vi "configure operation.vi"(7 "tag bus configurable plugin module configuration":refnum<class "Modbus Module configuration.lvclass">, 8 "error in":errorcluster, 10 "line item in":T2, 11 "engine configuration":refnum<class "engine configuration.lvclass">) -> (0 "error out":errorcluster, 1 "success":bool, 2 "line item out":T2, 5 "changed":bool)   [LabVIEW 2013, in "Modbus Module editor node.lvclass"]
doc: "Platypus Framework 1.0.1.65\nNI Systems Engineering - National Instruments"
uses:
  Modbus Module editor node.lvclass
  permissions.ctl
  table line.ctl
  module/module channel/Modbus Module Channel.lvclass
  <vilib>/NI/Module Execution Interface/Engine Configuration/engine configuration.lvclass
  module/configuration/Modbus Module configuration.lvclass
  module/module channel/data bank type.ctl
  <vilib>/NI/Tag Bus/tag/tag descriptor.lvclass/tag descriptor.ctl
  <vilib>/NI/Tag Bus Module Framework/channel/TBM channel.lvclass/TBM channel.ctl
  module/module channel/Modbus Module Channel.lvclass/Modbus Module Channel.ctl
  <vilib>/NI/Configuration Framework/serializable configuration/NISE_CEF_serializable configuration.lvclass/NISE_CEF_serializable configuration.ctl
  <vilib>/NI/Tag Bus/tag/Data Type.ctl
  <vilib>/NI/Tag Bus Module Framework/channel/Read channel classification.vi
  module/module channel/Read modbus type.vi
  module/module channel/Read starting address.vi
  module/module channel/Read subindex (bool).vi
  <vilib>/NI/Tag Bus/tag/read data type.vi
  <vilib>/NI/Configuration Framework/serializable configuration/Read UID.vi
  <vilib>/NI/Tag Bus/tag/write data type.vi
  <vilib>/NI/Tag Bus Module Framework/channel/Write channel classification.vi
  module/module channel/Write modbus type.vi
  module/module channel/Write starting address.vi
  module/module channel/Write subindex (bool).vi
  <vilib>/NI/Tag Bus/tag/write tag name.vi
  <vilib>/Utility/LVClass/Get LV Class Name.vi
  <vilib>/NI/Configuration Framework/error generator/NISE_error generator.vi
  <vilib>/NI/Tag Bus/tag/tag descriptor.lvclass
panel:
  in  "Channel Name":string
  out "Alias":string
  out "issues":string
  in  "Tag":i32(listbox)
  in  "Type":i32(listbox)
  in  "Bit/Length":i32 min=0 max=15 step=1
  in  "Address (0 index)":enum16{""}(ring)
  in  "modbus bank":T1
  in  "cancel":bool
  in  "ok":bool
  in  "Access Type":T3
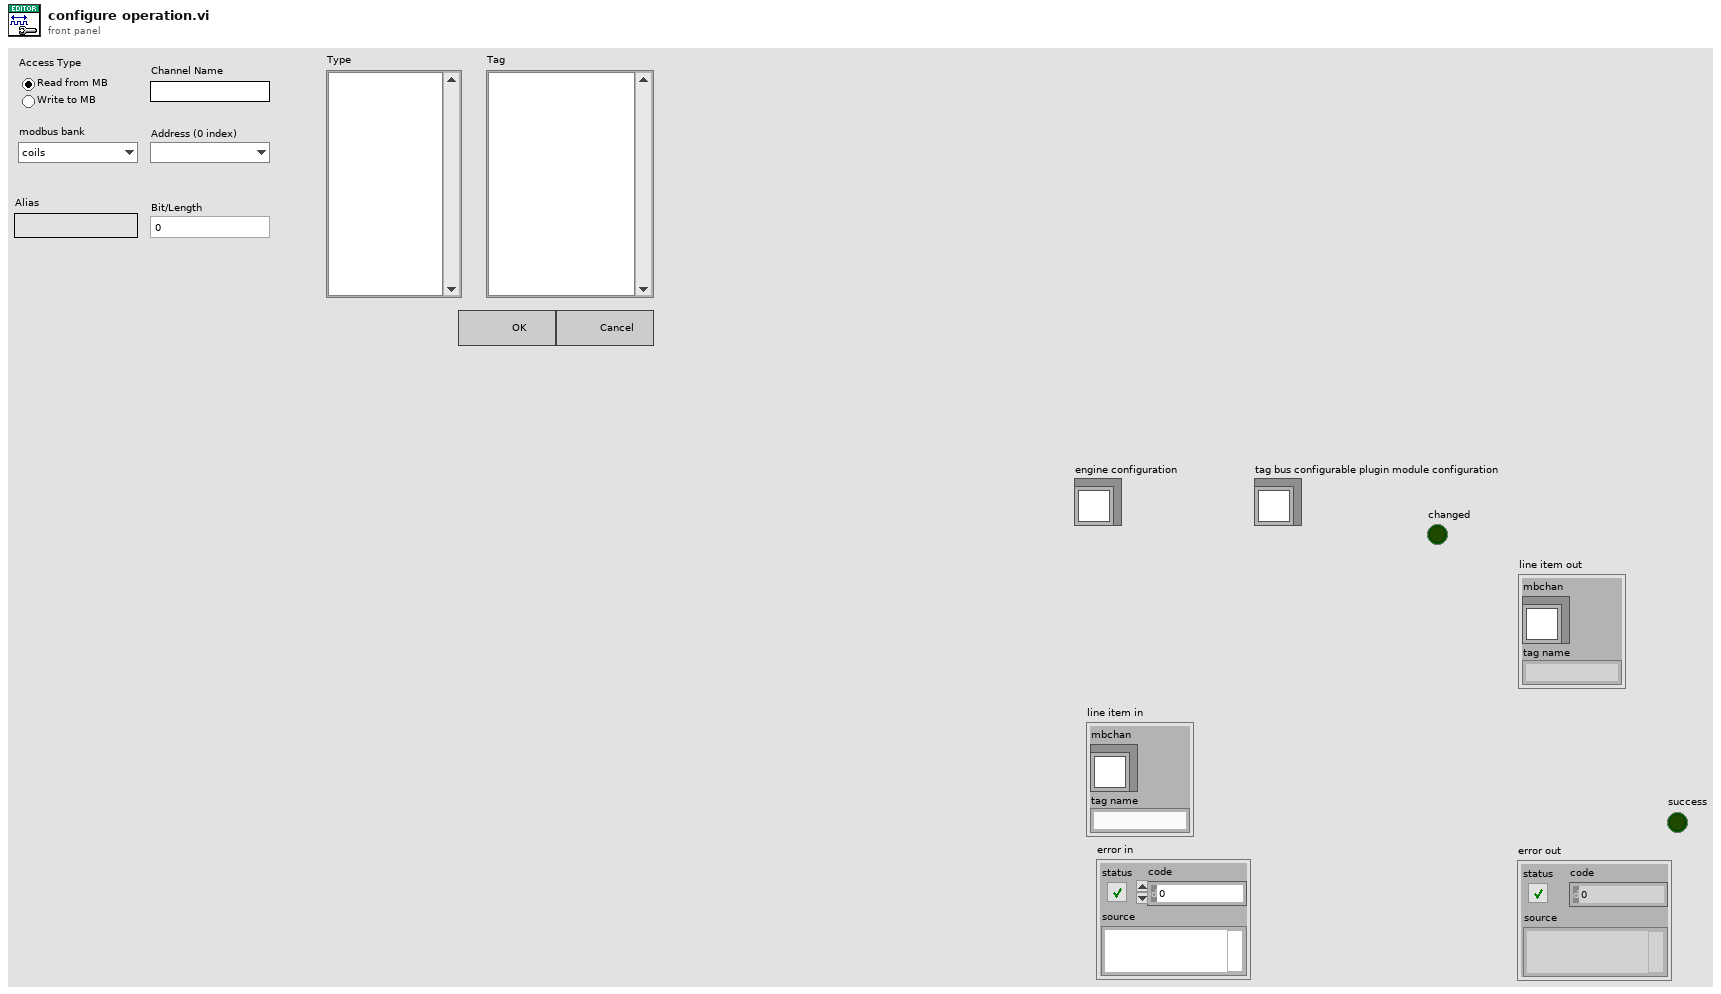
[diagram p1: front panel]
types:
  T1 = typedef "Modbus Module Channel.lvclass/data bank type.ctl" = enum16{"coils", "discrete inputs", "input registers", "holding registers"}
  T2 = typedef "Modbus Module editor node.lvclass/table line.ctl" = cluster{"mbchan":refnum<class "Modbus Module Channel.lvclass">, "tag name":string}
  T3 = typedef "Modbus Module editor node.lvclass/permissions.ctl" = enum32{"Read from MB", "Write to MB"}
  T4 = enum32{"Invalid", "Standard", "Closed", "Hidden", "Minimized", "Maximized"}
  T5 = enum32{"Invalid", "Default", "Floating", "Floating/Auto-Hide", "Modal"}
  T6 = enum8{"Enabled", "Disabled", "Disabled and Grayed Out"}
  T7 = typedef "tag bus.lvlib/tag descriptor.lvclass/Data Type.ctl" = enum16{"Double", "Single", "I64", "I32", "I16", "I8", "U64", "U32", "U16", "U8", "Boolean", "String", "Array of Double", "Array of Single", "Array of I64", "Array of I32", "Array of I16", "Array of I8", "Array of U64", "Array of U32", "Array of U16", "Array of U8", "Array of Boolean", "Array of String"}
  T8 = enum32{"invalid app kind", "Development System", "Run Time System", "Student Edition", "Embedded LabVIEW", "Evaluation", "Custom"}
  T9 = typedef "TBM channel.lvclass/channel classification.ctl" = enum16{"input data", "output data", "processing parameter", "processing result"}
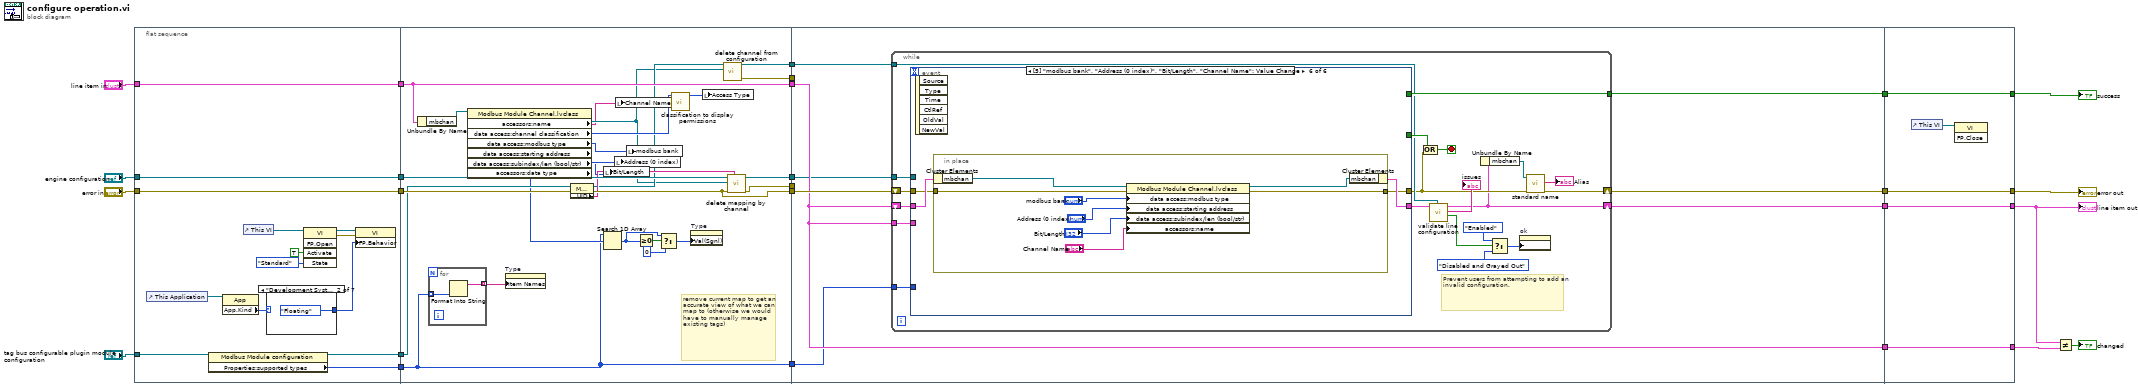
[diagram p0: block diagram]
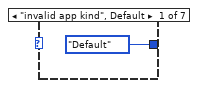
[diagram p2: hidden frame]
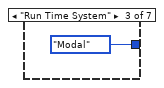
[diagram p3: hidden frame]
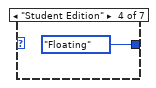
[diagram p4: hidden frame]
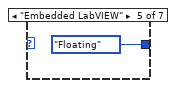
[diagram p5: hidden frame]
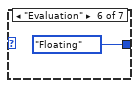
[diagram p6: hidden frame]
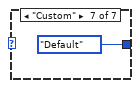
[diagram p7: hidden frame]
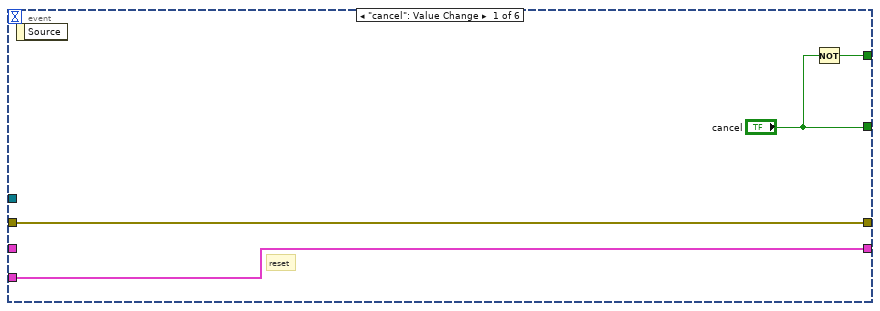
[diagram p8: hidden frame]
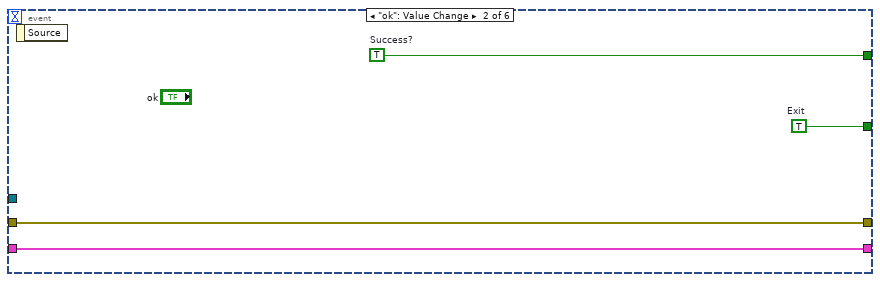
[diagram p9: hidden frame]
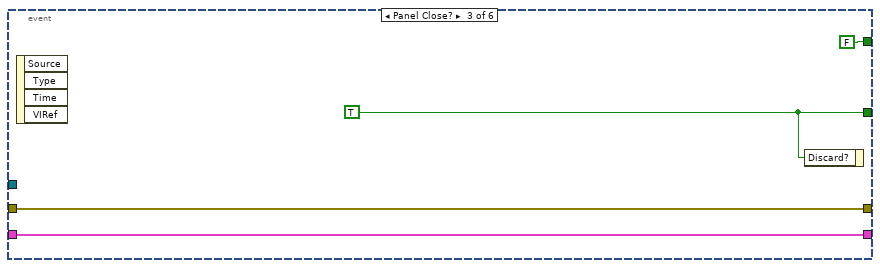
[diagram p10: hidden frame]
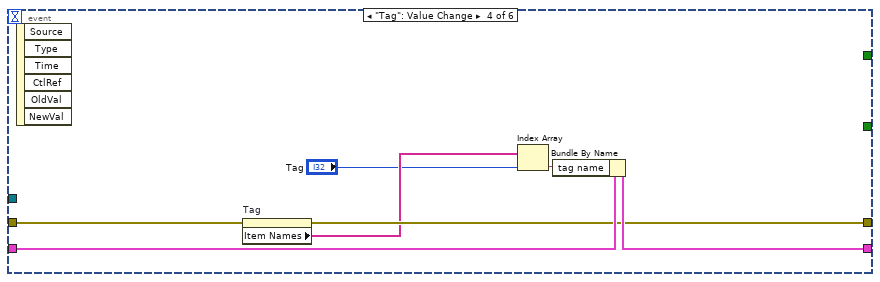
[diagram p11: hidden frame]
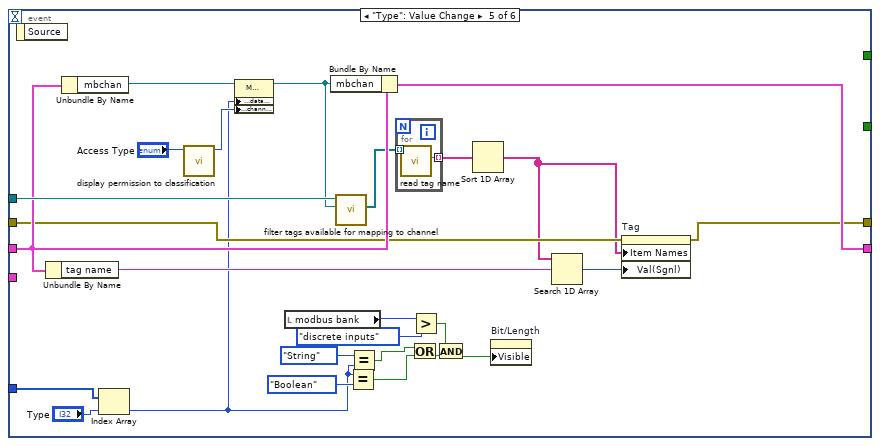
[diagram p12: hidden frame]
diagram:
  n1 = flat-sequence {
    tunnel: "line item in" -> [w38]
    tunnel: "error in" -> [w39]
    tunnel: [w39] -> w14
    tunnel: [w38] -> w13
    tunnel: [w29] -> w10
    tunnel: "engine configuration" -> [w29]
    tunnel: [w27] -> w8
    tunnel: "tag bus configurable plugin module configuration" -> [w28]
    tunnel: [w26] -> w4
    tunnel: w14 -> [w65]
    tunnel: w13 -> [w69]
    tunnel: [w69] -> w12
    tunnel: [w67] -> w11
    tunnel: w10 -> [w68]
    tunnel: w8 -> [w63]
    tunnel: [w64] -> w6
    tunnel: [w66] -> w5
    tunnel: w4 -> [w53]
    tunnel: [w53] -> w3
    tunnel: [w50] -> w2
    tunnel: [w49] -> w1
    tunnel: [w81] -> w18
    tunnel: [w80] -> w17
    tunnel: [w76] -> w16
    tunnel: [w79] -> w15
    tunnel: w12 -> [w79]
    tunnel: w11 -> [w78]
    tunnel: w6 -> [w82]
    tunnel: w5 -> [_]
    tunnel: w3 -> [w75]
    tunnel: w2 -> [w77]
    tunnel: w1 -> [_]
    tunnel: [w163] -> w19
    tunnel: [w164] -> w22
    tunnel: [w165] -> w23
    tunnel: [w166] -> w24
    tunnel: w18 -> [w166]
    tunnel: w17 -> [w165]
    tunnel: w16 -> [w164]
    tunnel: w15 -> [w163]
    frame #0 {
      n2 = control-ref of="This Application"() -> (w32:refnum<vi>)
      n3 = property class="Modbus Module configuration"(reference=w28) -> (reference out=w27:refnum<class "Modbus Module configuration.lvclass">, "Properties:supported types"=w26:T7[])  [unwired: 1 in, 1 out]
      n4 = property class="App"(reference=w32) -> ("App.Kind"=w31:T8)  [unwired: 1 in, 2 out]
      n5 = control-ref of="This VI"() -> (w33:refnum<vi>)
      n6 = case shown="\"Development System\"" w31 {
        tunnel: [T5."Default" ("Front Panel Window:Behavior") T5."Floating" ("Front Panel Window:Behavior") T5."Modal" ("Front Panel Window:Behavior") T5."Floating" ("Front Panel Window:Behavior") T5."Floating" ("Front Panel Window:Behavior") T5."Floating" ("Front Panel Window:Behavior") T5."Default" ("Front Panel Window:Behavior")] -> w30
        frame "invalid app kind", Default {
        }
        frame "Development System" {
        }
        frame "Run Time System" {
        }
        frame "Student Edition" {
        }
        frame "Embedded LabVIEW" {
        }
        frame "Evaluation" {
        }
        frame "Custom" {
        }
      }
      n7 = invoke class="VI" method="FP.Open"(reference=w33, "Activate"=TRUE ("Activate?"), "State"=T4."Standard") -> (reference out=w36:refnum<vi>, error out=w37:errorcluster)  [unwired: 2 in, 3 out]
      n8 = property class="VI"(reference=w36, error in=w37, "FP.Behavior"=w30) -> ()  [unwired: 2 out]
    }
    frame #1 {
      # "remove current map to get an accurate view of what we can map to (otherwise we would have to manually manage existing tags)"
      n9 = Unbundle By Name(w69) -> ("mbchan"=w71:refnum<class "Modbus Module Channel.lvclass">)
      n10 = for {
        tunnel: w53 -> [w74] mode=indexing
        tunnel: [w73] -> w52 mode=indexing
        n11 = Format Into String(w74) -> (resulting string=w73:string)  [unwired: 3 in, 1 out]
      }
      n12 = property class="Modbus Module Channel.lvclass"(reference=w71) -> (reference out=w48:refnum<class "Modbus Module Channel.lvclass">, "accessors:name"=w47:string, "data access:channel classification"=w72:T9, "data access:modbus type"=w61:T1, "data access:starting address"=w60:u16, "data access:subindex/len (bool/str)"=w59:i32, "accessors:data type"=w58:T7)  [unwired: 1 in, 1 out]
      n13 = property on="Type" class="LstBox (strict)"("Item Names"=w52) -> ()  [unwired: 2 in, 2 out]
      n14 = property class="Modbus Module configuration"(reference=w63, error in=w65) -> (reference out=w51:refnum<class "Modbus Module configuration.lvclass">, error out=w64:errorcluster, "Properties:UID"=w62:string)
      n15 = local write "Bit/Length"(w59) -> ()
      n16 = Search 1D Array(1D array=w53, element=w58) -> (index of element=w55:i32)  [unwired: 1 in]
      n17 = local write "Address (0 index)"(w60) -> ()
      n18 = local write "Channel Name"(w47) -> ()
      n19 = local write "modbus bank"(w61) -> ()
      n20 = Greater Or Equal To 0?(x=w55) -> (x >= 0?=w57:bool)
      n21 = Select(t=w55, s=w57, f=0) -> (s? t:f=w56:i32)
      n22 = call "classification to display permissions.vi"("channel classification"=w72) -> ("permissions"=w70:T3)  [unwired: 10 in]
      n23 = property on="Type" class="LstBox (strict)"("Val(Sgnl)"=w56) -> ()  [unwired: 2 in, 2 out]
      n24 = local write "Access Type"(w70) -> ()
      n25 = call "delete channel from configuration.vi"("Modbus Module Channel.lvclass"=w48, "Modbus Slave configuration in"=w51) -> ("error out"=w49:errorcluster, "Modbus Slave configuration out"=w50:refnum<class "Modbus Module configuration.lvclass">)  [unwired: 8 in]
      n26 = call <vilib>:"delete mapping by channel.vi"("owner ID"=w62, "error in"=w64, "channel"=w48, "engine configuration in"=w68) -> ("error out"=w66:errorcluster, "engine configuration out"=w67:refnum<class "engine configuration.lvclass">)  [unwired: 6 in]
    }
    frame #2 {
      n27 = while {
        shift-right: [w87] -> w80
        shift-left: w82 -> [w101]
        tunnel: [w100] -> w81
        shift-right: [w85] -> w76
        shift-left: w79 -> [w97]
        tunnel: w79 -> [w96]
        tunnel: w78 -> [w102]
        tunnel: w77 -> [w90]
        tunnel: w75 -> [w89]
        stop <- w98 stop-if-true
        # "Prevent users from attempting to add an invalid configuration."
        n28 = event shown="[5] \"modbus bank\", \"Address (0 index)\", \"Bit/Length\", \"Channel Name\": Value Change" {
          selector: _ -> [_ _ _ _ _ _]
          dyn-events: _ -> [_ _ _ _ _ _]
          timeout: _ -> [_ _ _ _ _ _]
          tunnel: w102 -> [_ _ _ _ w144 _]
          tunnel: w101 -> [w106 w110 w114 w118 w130 w151]
          tunnel: [w106 w110 w114 w117 w129 w150] -> w86
          tunnel: [w105 w107 FALSE _ _ _] -> w100
          tunnel: ["cancel" w108 w112 _ _ _] -> w99
          tunnel: w97 -> [_ w109 w111 w121 w142 w153]
          tunnel: [w103 w109 w111 w120 w133 w152] -> w95
          tunnel: w96 -> [w103 _ _ _ _ _]
          tunnel: w89 -> [_ _ _ _ w127 _]
          event "cancel": Value Change {
            # "reset"
            n29 = event-data() -> ()  [unwired: 1 in, 1 out]
            n30 = Not(x="cancel") -> (.not. x?=w105:bool)
          }
          event "ok": Value Change {
            w107 = TRUE  # Success?
            w108 = TRUE  # Exit
            n31 = event-data() -> ()  [unwired: 1 in, 1 out]
          }
          event Panel Close? {
            w112 = TRUE ("cancel")
            n32 = event-data() -> ()  [unwired: 1 in, 4 out]
            n33 = event-data("Discard?"=w112) -> ()  [unwired: 1 in, 1 out]
          }
          event "Tag": Value Change {
            n34 = event-data() -> ()  [unwired: 1 in, 6 out]
            n35 = property on="Tag" class="LstBox (strict)"(error in=w118) -> (error out=w117:errorcluster, "Item Names"=w116:string[])  [unwired: 1 in, 1 out]
            n36 = Index Array(array=w116, index="Tag") -> (element=w119:string)
            n37 = Bundle By Name(cluster=w121, "tag name"=w119) -> (w120:T2)
          }
          event "Type": Value Change {
            n38 = event-data() -> ()  [unwired: 1 in, 1 out]
            n39 = Unbundle By Name(w142) -> ("tag name"=w134:string)
            n40 = Unbundle By Name(w142) -> ("mbchan"=w146:refnum<class "Modbus Module Channel.lvclass">)
            n41 = Index Array(array=w127, index="Type") -> (element=w125:T7)
            n42 = call "display permission to classification.vi"("display permissions"="Access Type") -> ("channel classification"=w145:T9)  [unwired: 10 in]
            n43 = property class="Modbus Module Channel.lvclass"(reference=w146, "accessors:data type"=w125, "data access:channel classification"=w145) -> (reference out=w143:refnum<class "Modbus Module Channel.lvclass">)  [unwired: 1 in, 1 out]
            n44 = local read "modbus bank"() -> (w138:T1)
            n45 = Bundle By Name(cluster=w142, "mbchan"=w143) -> (w133:T2)
            n46 = call <vilib>:"filter tags available for mapping to channel.vi"("channel to map to"=w143, "engine configuration in"=w144) -> ("filtered tags"=w141:refnum<class "tag descriptor.lvclass">[])  [unwired: 8 in, 1 out]
            n47 = Equal?(x=w125, y=Data_Type."Boolean") -> (x = y?=w139:bool)
            n48 = Equal?(x=Data_Type."String", y=w125) -> (x = y?=w123:bool)
            n49 = for {
              tunnel: w141 -> [w149] mode=indexing
              tunnel: [w148] -> w131 mode=indexing
              n50 = call <vilib>:"read tag name.vi"("system tag in"=w149) -> ("name"=w148:string)  [unwired: 8 in, 2 out]
            }
            n51 = Or(x=w123, y=w139) -> (x .or. y?=w126:bool)
            n52 = Greater?(x=w138, y=data_bank_type."discrete inputs") -> (0:w135:bool)
            n53 = And(x=w135, y=w126) -> (x .and. y?=w136:bool)
            n54 = Sort 1D Array(array=w131) -> (sorted array=w122:string[])
            n55 = property on="Bit/Length" class="DigNum (strict)"("Visible"=w136) -> ()  [unwired: 2 in, 2 out]
            n56 = Search 1D Array(1D array=w122, element=w134) -> (index of element=w132:i32)  [unwired: 1 in]
            n57 = property on="Tag" class="LstBox (strict)"(error in=w130, "Item Names"=w122, "Val(Sgnl)"=w132) -> (error out=w129:errorcluster)  [unwired: 1 in, 1 out]
          }
          event "Address (0 index)", "Bit/Length", "Channel Name": Value Change {
            n58 = event-data() -> ()  [unwired: 1 in, 6 out]
            n59 = in-place {
              in-place-border: w151 -> [w161]
              in-place-border: [w155] -> w150
              n60 = in-place-cluster #1(w153) -> ("mbchan"=w160:refnum<class "Modbus Module Channel.lvclass">)
              n61 = property class="Modbus Module Channel.lvclass"(reference=w160, error in=w161, "data access:modbus type"="modbus bank", "data access:starting address"="Address (0 index)", "data access:subindex/len (bool/str)"="Bit/Length", "accessors:name"="Channel Name") -> (reference out=w156:refnum<class "Modbus Module Channel.lvclass">, error out=w155:errorcluster)
              n62 = in-place-cluster #1("mbchan"=w156) -> (w152:T2)
            }
          }
        }
        n63 = Compound Arithmetic op=OR(w99, w86) -> (w98:bool)
        n64 = call "validate line configuration.vi"("modbus"=w90, "line in"=w95) -> ("valid?"=w94:bool, "issues"=→"issues":string, "line out"=w85:T2)  [unwired: 7 in]
        n65 = Unbundle By Name(w85) -> ("mbchan"=w84:refnum<class "Modbus Module Channel.lvclass">)
        n66 = Select(t=T6."Enabled" ("Disabled"), s=w94, f=T6."Disabled and Grayed Out") -> (s? t:f=w91:T6)
        n67 = property on="ok" class="Bool"("DisabledEnum"=w91) -> ()  [unwired: 2 in, 2 out]
        n68 = call "standard name.vi"("error in"=w86, "Modbus Module Channel in"=w84) -> ("error out"=w87:errorcluster, "standard name"=→"Alias":string)  [unwired: 7 in, 1 out]
      }
    }
    frame #3 {
      n69 = control-ref of="This VI"() -> (w162:refnum<vi>)
      n70 = invoke class="VI" method="FP.Close"(reference=w162) -> ()  [unwired: 2 in, 3 out]
    }
  }
  n71 = Not Equal?(x=w22, y=w19) -> (x != y?=→"changed":bool)
  "error out" <- w23
  "success" <- w24
  "line item out" <- w22
